vi "svc_Reshape Waveform into Array of Waveform Subsets.vi"(7 "restart":bool, 9 "block size (s)":dbl, 11 "block in":waveform(dbl)) -> (1 "number of blocks":i32, 3 "block(s) out":waveform(dbl)[](array[waveform]))   [LabVIEW 2017]
uses:
  <vilib>/Waveform/WDTOps.llb/WDT Get Waveform Subset DBL.vi
  <vilib>/Waveform/WDTOps.llb/WDT Append Waveforms DBL.vi
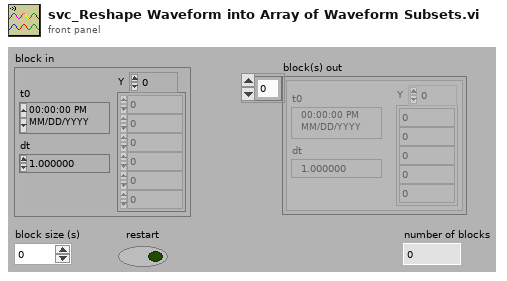
[diagram p1: front panel]
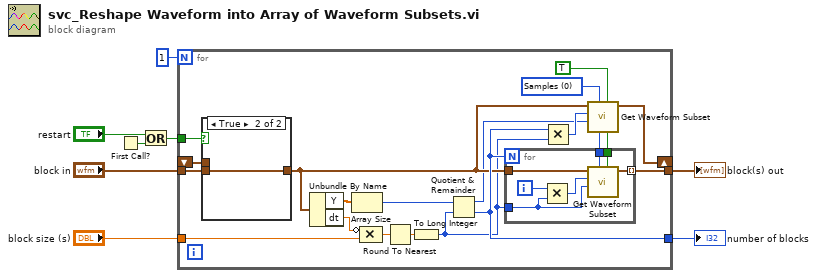
[diagram p0: block diagram]
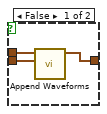
[diagram p2: hidden frame]
diagram:
  n1 = First Call?() -> (First Call?: T/F=w5:bool)
  n2 = Or(x="restart", y=w5) -> (x .or. y?=w1:bool)
  n3 = for {
    N: 1 -> [_]
    tunnel: "block size (s)" -> [w18]
    shift-right: [w21] -> _
    shift-left: _ -> [w26]
    tunnel: [w25] -> w8
    tunnel: "block in" -> [w19]
    tunnel: [w12] -> w3
    tunnel: w1 -> [w24]
    w22 = TRUE ("open interval? (T)")
    w23 = u16 0 items=["Samples", "Relative Time"] ("start/duration format")
    n4 = case shown="True" w24 {
      tunnel: w26 -> [w35 _]
      tunnel: w19 -> [w36 w37]
      tunnel: [w34 w37] -> w11
      frame False {
        n5 = call-poly <vilib>:"Append Waveforms.vi"("waveform B"=w36, "waveform A"=w35) -> ("waveform out"=w34:waveform(dbl))  [unwired: 8 in, 1 out]
      }
      frame True {
      }
    }
    n6 = Unbundle By Name(w11) -> ("Y"=w17:dbl[], "dt"=w15:dbl)
    n7 = Array Size(array=w17) -> (size(s)=w16:i32)
    n8 = Compound Arithmetic op=MULTIPLY(invert w15, w18) -> (w14:dbl)
    n9 = Round To Nearest(number=w14) -> (nearest integer value=w13:dbl)
    n10 = To Long Integer(number=w13) -> (32bit integer=w10:i32)
    n11 = Quotient & Remainder(x=w16, y=w10) -> (x-y*floor(x/y)=w9:i32, floor(x/y)=w12:i32)
    n12 = for {
      N: w12 -> [_]
      tunnel: w11 -> [w33]
      tunnel: w23 -> [w32]
      tunnel: w10 -> [w27]
      tunnel: [w30] -> w25 mode=indexing
      tunnel: w22 -> [w29]
      i -> [w31]
      n13 = Multiply(x=w31, y=w27) -> (x*y=w28:i32)
      n14 = call-poly <vilib>:"Get Waveform Subset.vi"("open interval? (T)"=w29, "start/duration format"=w32, "duration"=w27, "start samples/time"=w28, "waveform in"=w33) -> ("waveform out"=w30:waveform(dbl))  [unwired: 1 in, 3 out]
    }
    n15 = Multiply(x=w12, y=w10) -> (x*y=w20:i32)
    n16 = call-poly <vilib>:"Get Waveform Subset.vi"("open interval? (T)"=w22, "start/duration format"=w23, "duration"=w9, "start samples/time"=w20, "waveform in"=w11) -> ("waveform out"=w21:waveform(dbl))  [unwired: 1 in, 3 out]
  }
  "block(s) out" <- w8
  "number of blocks" <- w3
